vi "Default Repo.vi"(1 "Repo in":string) -> (0 "Repo out":string)   [LabVIEW 2019, in "SelfUpdate.lvclass"]
uses:
  SelfUpdate.lvclass
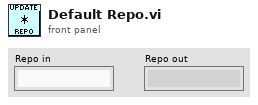
[diagram p1: front panel]
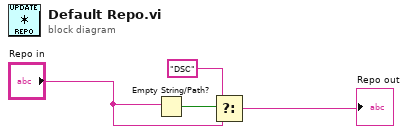
[diagram p0: block diagram]
diagram:
  n1 = Empty String/Path?(string/path="Repo in") -> (empty?=w1:bool)
  n2 = Select(t="DSC", s=w1, f="Repo in") -> (s? t:f=→"Repo out":string)
